vi "GetLocalComputerName.vi"(8 "error in (no error)":errorcluster) -> (0 "error out":errorcluster, 1 "Full Name":string, 2 "Name":string)   [LabVIEW 2016]
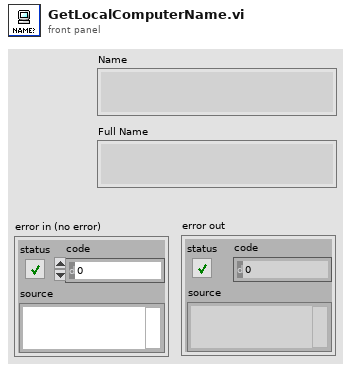
[diagram p1: front panel]
types:
  T1 = typedef "Dictionary Object RefNum__ogtk.ctl" = refnum<k1>
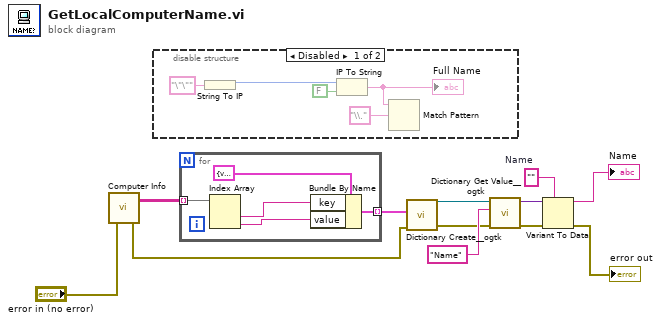
[diagram p0: block diagram]
diagram:
  w5 = ""  # Name
  n1 = call "Computer Info.vi"("error in (no error)"="error in (no error)") -> ("error out"=w3:errorcluster, "Computer Info"=w12:string[][])  [unwired: 1 in]
  n2 = disable-structure shown="Disabled" {
    frame Disabled {
      n3 = String To IP(1:"\"\"" ("name")) -> (0:w16:u32)
      n4 = IP To String(1:FALSE ("dot notation? (F)"), 2:w16) -> (0:w13:string)
      "Full Name" <- w13
      n5 = Match Pattern(string=w13, regular expression="\\.") -> ()  [unwired: 1 in, 4 out]
    }
    frame Enabled {
    }
  }
  n6 = for {
    tunnel: w12 -> [w22] mode=indexing
    tunnel: [w18] -> w11 mode=indexing
    n7 = Index Array(array=w22) -> (element #1=w20:string, element #2=w19:string)  [unwired: 2 in]
    n8 = Bundle By Name(cluster=cluster{"key":variant, "value":variant} {"key"=variant, "value"=variant} ("key-value"), "key"=w20, "value"=w19) -> (w18:cluster{"key":variant, "value":variant})
  }
  n9 = call <userlib>:"Dictionary Create__ogtk.vi"("error in (no error)"=w3, "initial dictionary (empty)"=w11) -> ("error out"=w8:errorcluster, "dictionary out"=w10:T1)  [unwired: 8 in]
  n10 = call <userlib>:"Dictionary Get Value__ogtk.vi"("error in"=w8, "key"="Name" ("element"), "dictionary"=w10) -> ("error out"=w7:errorcluster, "value"=w6:variant)  [unwired: 5 in, 2 out]
  n11 = Variant To Data(error in=w7, type=w5, Variant=w6) -> (data=→"Name":string, error out=→"error out":errorcluster)
